vi "emi_Write Key Anything.vi"(0 "Ini file refnum":T1, 1 "Section(Default)":string="Default", 5 "Name":string, 7 "Anything":variant, 11 "error in (no error)":errorcluster) -> (4 "Ini file refnum out":T1, 15 "error out":errorcluster)   [LabVIEW 2011]
doc: "Use in the same way as Read key. Anything in may contain a cluster.\nAny data wired to Anything must be named, that includes any item in a cluster.\nThis is a slow VI, keep in mind when desiding where to use.\n\nARRAY SUPPIORT FUNKER IKKE. \n\nThe cluster can contain anything(Including other clusters) except:\nARRAY\nVariant\nPicture\nTag\nWaveform\nDigital Waveform\nDigital Data\nExpressData\nRefnum\nExternal Data\nVI\nPoly VI\nLabview Class Instance\nFixed point\n\nOn Error: No operation"
uses:
  <vilib>/Utility/config.llb/Config Data RefNum.ctl
  Error/emi_Create Error.vi
  <vilib>/Utility/VariantDataType/GetNumericInfo.vi
  <vilib>/Utility/config.llb/Write Key (String).vi
  <vilib>/Utility/VariantDataType/VariantType.lvlib
  <vilib>/Utility/config.llb/NI_LVConfig.lvlib
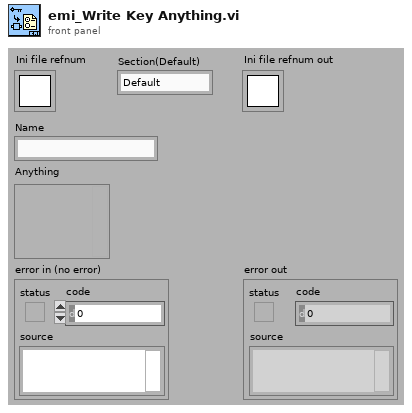
[diagram p1: front panel]
types:
  T1 = typedef "NI_LVConfig.lvlib/Config Data RefNum.ctl" = refnum<k1>
  T2 = typedef "VariantType.lvlib/Type.ctl" = enum8{"Invalid Type", "Void", "I8", "I16", "I32", "I64", "U8", "U16", "U32", "U64", "Single Float", "Double Float", "Extended Float", "Single Complex", "Double Complex", "Extended Complex", "Enum U8", "Enum U16", "Enum U32", "Enum U64", "Single Float With Unit", "Double Float With Unit", "Extended Float With Unit", "Single Complex with Unit", "Double Complex with Unit", "Extended Complex with Unit", "Boolean", "String", "Path", "Picture", "Tag", "Array", "Cluster", "Variant", "LV Variant", "Waveform", "Timestamp", "Digital Waveform", "Digital Data", "ExpressData", "Refnum", "External Data", "VI", "Poly VI", "LabVIEW Class Instance", "Fixed Point"}
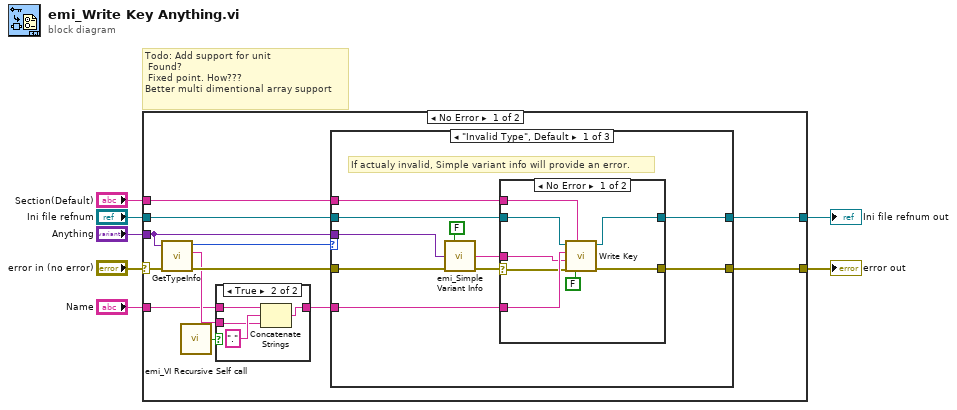
[diagram p0: block diagram]
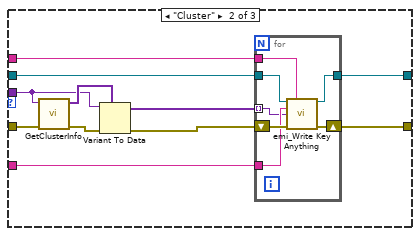
[diagram p3: hidden frame]
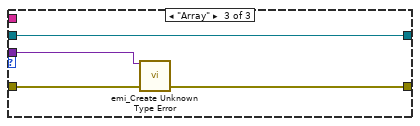
[diagram p4: hidden frame]
diagram:
  # "Todo: Add support for unit\n Found?\n Fixed point. How???\nBetter multi dimentional array support"
  n1 = case shown="No Error" "error in (no error)" {
    selector: "error in (no error)" -> [w16 w68]
    tunnel: "Anything" -> [w18 _]
    tunnel: [w15 w68] -> w5
    tunnel: "Name" -> [w13 _]
    tunnel: "Ini file refnum" -> [w11 w67]
    tunnel: "Section(Default)" -> [w10 _]
    tunnel: [w9 w67] -> w1
    frame No Error {
      n2 = call <vilib>:"GetTypeInfo.vi"("error in (no error)"=w16, "Variant"=w18) -> ("error out"=w17:errorcluster, "Name"=w14:string, "Type Enum"=w19:T2)  [unwired: 5 in, 2 out]
      n3 = call "emi_VI Recursive Self call.vi"() -> ("Recursive Self Call?"=w8:bool)  [unwired: 15 in]
      n4 = case shown="True" w8 {
        tunnel: w14 -> [_ w65]
        tunnel: w13 -> [w62 w64]
        tunnel: [w62 w63] -> w12
        frame False {
        }
        frame True {
          n5 = Concatenate Strings(w64, "." ("string"), w65) -> (w63:string)
        }
      }
      n6 = case shown="\"Invalid Type\", Default" w19 {
        tunnel: w18 -> [w29 w41 w58]
        tunnel: w17 -> [w28 w45 w59]
        tunnel: [w27 w46 w60] -> w15
        tunnel: w12 -> [w25 w48 _]
        tunnel: w10 -> [w24 w49 _]
        tunnel: w11 -> [w26 w50 w61]
        tunnel: [w23 w47 w61] -> w9
        frame "Invalid Type", Default {
          # "If actualy invalid, Simple variant info will provide an error."
          n7 = call "emi_Simple Variant Info.vi"("use system decimal point (T)"=FALSE, "Anything"=w29, "error in(no error)"=w28) -> ("String Value"=w22:string, "error out"=w21:errorcluster)  [unwired: 9 in, 2 out]
          n8 = case shown="No Error" w21 {
            selector: w21 -> [w31 w39]
            tunnel: [w37 w39] -> w27
            tunnel: w26 -> [w36 w38]
            tunnel: w25 -> [w35 _]
            tunnel: w24 -> [w34 _]
            tunnel: [w33 w38] -> w23
            tunnel: w22 -> [w32 _]
            frame No Error {
              n9 = call-poly <vilib>:"Write Key.vi"("write raw string? (F)"=FALSE, "section"=w34, "error in (no error)"=w31, "value"=w32, "key"=w35, "refnum"=w36) -> ("error out"=w37:errorcluster, "refnum out"=w33:T1)  [unwired: 3 in, 1 out]
            }
            frame Error {
            }
          }
        }
        frame "Cluster" {
          n10 = call <vilib>:"GetClusterInfo.vi"("error in (no error)"=w45, "Variant"=w41) -> ("error out"=w44:errorcluster, "Cluster Elements"=w42:variant[])  [unwired: 8 in]
          n11 = Variant To Data(error in=w44, type=w42, Variant=w41) -> (data=w40:variant[], error out=w43:errorcluster)
          n12 = for {
            tunnel: w40 -> [w51] mode=indexing
            tunnel: w48 -> [w52]
            tunnel: w50 -> [w55]
            tunnel: w49 -> [w54]
            tunnel: [w53] -> w47
            shift-right: [w56] -> w46
            shift-left: w43 -> [w57]
            n13 = call "emi_Write Key Anything.vi"("Ini file refnum"=w55, "Section(Default)"=w54, "Name"=w52, "Anything"=w51, "error in (no error)"=w57) -> ("Ini file refnum out"=w53:T1, "error out"=w56:errorcluster)  [unwired: 9 in]
          }
        }
        frame "Array" {
          n14 = call "emi_Create Unknown Type Error.vi"("Anything"=w58, "error IO"=w59) -> ("error out"=w60:errorcluster)  [unwired: 13 in]
        }
      }
    }
    frame Error {
    }
  }
  "error out" <- w5
  "Ini file refnum out" <- w1
